vi "AutoFollowAbsoluteTrajectoryNEW.vi"(8 "error in (no error)":errorcluster, 9 "TimeOut (s)":dbl, 10 "End Orientation":dbl, 11 "Trajectory":T1 {"States"."POSE"."ROTATION"."SIN" format="%13.4f"; "States"."POSE"."ROTATION"."COS" format="%13.4f"; "States"."POSE"."ROTATION"."VALUE" format="%13.4f"; "States"."POSE"."TRANSLATION"."Y" format="%14.3f"; "States"."POSE"."TRANSLATION"."X" format="%14.3f"; "TotalTImeSecs" format="%20.3f"}) -> (0 "error out":errorcluster)   [LabVIEW 2023]
doc: "Wrapper class for drive straight"
uses:
  <vilib>/Rock Robotics/WPI/ThirdParty/JAS_Junk/TrajLib/Trajectory_Library.lvlib
  <vilib>/Rock Robotics/WPI/ThirdParty/JAS_Junk/TrajLib/TypeDef/TRANSLATION2D.ctl
  <vilib>/Rock Robotics/WPI/ThirdParty/JAS_Junk/TrajLib/TypeDef/ROTATION2D.ctl
  <vilib>/Rock Robotics/WPI/ThirdParty/JAS_Junk/TrajLib/TypeDef/POSE2D.ctl
  <vilib>/Rock Robotics/WPI/ThirdParty/JAS_Junk/TrajLib/TypeDef/TRAJ_STATE.ctl
  <vilib>/Rock Robotics/WPI/ThirdParty/JAS_Junk/TrajLib/TypeDef/TRAJECTORY.ctl
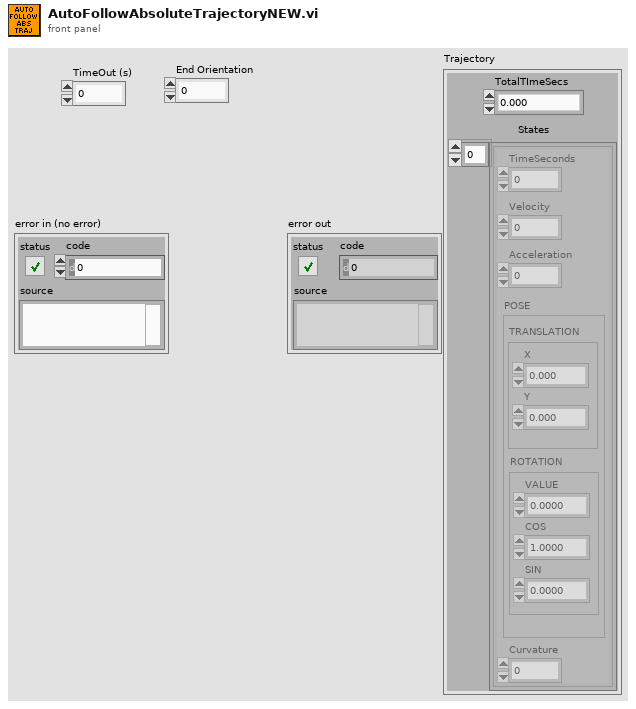
[diagram p1: front panel]
types:
  T1 = typedef "Trajectory_Library.lvlib/TRAJECTORY.ctl" = cluster{"TotalTImeSecs":dbl, "States":T2[]}
  T2 = typedef "Trajectory_Library.lvlib/TRAJ_STATE.ctl" = cluster{"TimeSeconds":dbl, "Velocity":dbl, "Acceleration":dbl, "POSE":T3, "Curvature":dbl}
  T3 = typedef "Trajectory_Library.lvlib/POSE2D.ctl" = cluster{"TRANSLATION":T4, "ROTATION":T5}
  T4 = typedef "Trajectory_Library.lvlib/TRANSLATION2D.ctl" = cluster{"X":dbl, "Y":dbl}
  T5 = typedef "Trajectory_Library.lvlib/ROTATION2D.ctl" = cluster{"VALUE":dbl, "COS":dbl, "SIN":dbl}
  T6 = typedef "Trajectory_Library.lvlib/TIMER.ctl" = cluster{"StartTime":dbl, "Accumulated TIme":dbl, "Running":bool, "semaphore":T7}
  T7 = typedef "Semaphore RefNum" = refnum<k1>
  T8 = typedef "Trajectory_Library.lvlib/CHASSIS_SPEEDS.ctl" = cluster{"vX":dbl, "vY":dbl, "vOmega":dbl}
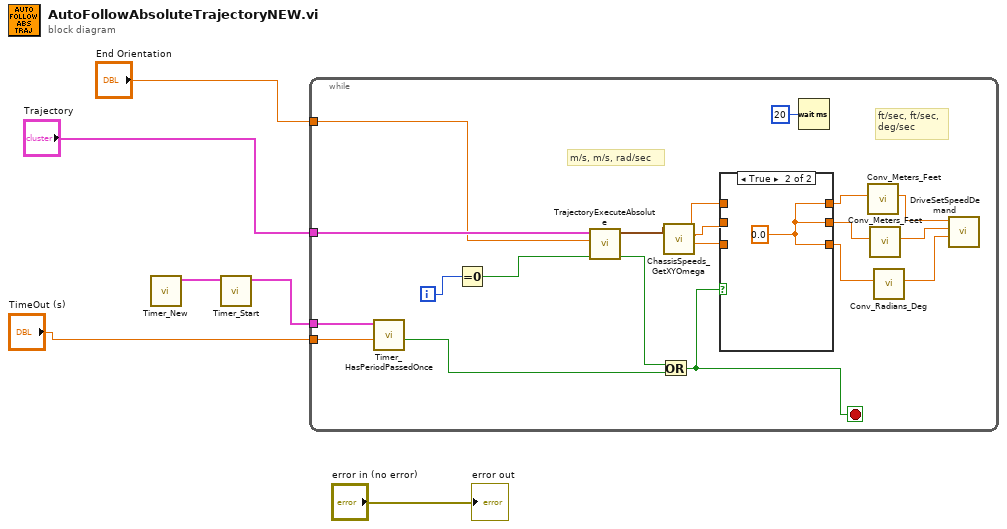
[diagram p0: block diagram]
diagram:
  n1 = call <vilib>:"Timer_New.vi"() -> ("TIMER"=w5:T6)  [unwired: 11 in]
  n2 = call <vilib>:"Timer_Start.vi"("in Timer"=w5) -> ("out Timer"=w4:T6)  [unwired: 10 in]
  n3 = while {
    tunnel: w4 -> [w25]
    tunnel: "TimeOut (s)" -> [w24]
    tunnel: "Trajectory" -> [w8]
    tunnel: "End Orientation" -> [w7]
    i -> [w26]
    stop <- w9 stop-if-true
    # "ft/sec, ft/sec,\ndeg/sec"
    # "m/s, m/s, rad/sec"
    n4 = call <vilib>:"Timer_HasPeriodPassedOnce.vi"("Period"=w24, "in Timer"=w25) -> ("Expired"=w23:bool)  [unwired: 7 in, 2 out]
    n5 = Equal To 0?(x=w26) -> (x = 0?=w21:bool)
    n6 = call "TrajectoryExecuteAbsolute.vi"("Init"=w21, "End Abs\nOrientation Deg"=w7, "Trajectory"=w8) -> ("AtReference"=w20:bool, "Chassis Velocity Target"=w16:T8)  [unwired: 7 in]
    n7 = Or(x=w20, y=w23) -> (x .or. y?=w9:bool)
    n8 = call <vilib>:"ChassisSpeeds_GetXYOmega.vi"("CHASSIS"=w16) -> ("vAngular"=w19:dbl, "vY"=w18:dbl, "vX"=w17:dbl)  [unwired: 8 in]
    n9 = case shown="True" w9 {
      tunnel: w17 -> [w29 _]
      tunnel: w18 -> [w28 _]
      tunnel: w19 -> [w27 _]
      tunnel: [w29 w30] -> w15
      tunnel: [w28 w30] -> w13
      tunnel: [w27 w30] -> w11
      frame False {
      }
      frame True {
        w30 = 0.0 ("XSpeedDemand")
      }
    }
    n10 = Wait (ms)(milliseconds to wait=u32 20) -> ()  [unwired: 1 out]
    n11 = call <vilib>:"Conv_Meters_Feet.vi"("Meters"=w15) -> ("Feet"=w14:dbl)  [unwired: 10 in]
    n12 = call <vilib>:"Conv_Meters_Feet.vi"("Meters"=w13) -> ("Feet"=w12:dbl)  [unwired: 10 in]
    n13 = call <vilib>:"Conv_Radians_Deg.vi"("Radians"=w11) -> ("Degrees"=w10:dbl)  [unwired: 10 in]
    n14 = call "DriveSetSpeedDemand.vi"("ASpeedDemand (d/s)"=w10, "YSpeedDemand (ft/s)"=w12, "XSpeedDemand (ft/s)"=w14) -> ()  [unwired: 9 in]
  }
  "error out" <- "error in (no error)"
